vi "anchor map.vi"(11 "string":string) -> (1 "Archt Map":variant, 3 "Lines":string[](array[string]))   [LabVIEW 2020, in "CSMStand-Engine(Lite).lvlib"]
uses:
  CSMStand-Engine(Lite).lvlib
  <userlib>/_NEVSTOP/Communicable State Machine(CSM)/_Shared/CSM Shared.lvlib
  <userlib>/_NEVSTOP/Communicable State Machine(CSM)/Communicable State Machine.lvlib
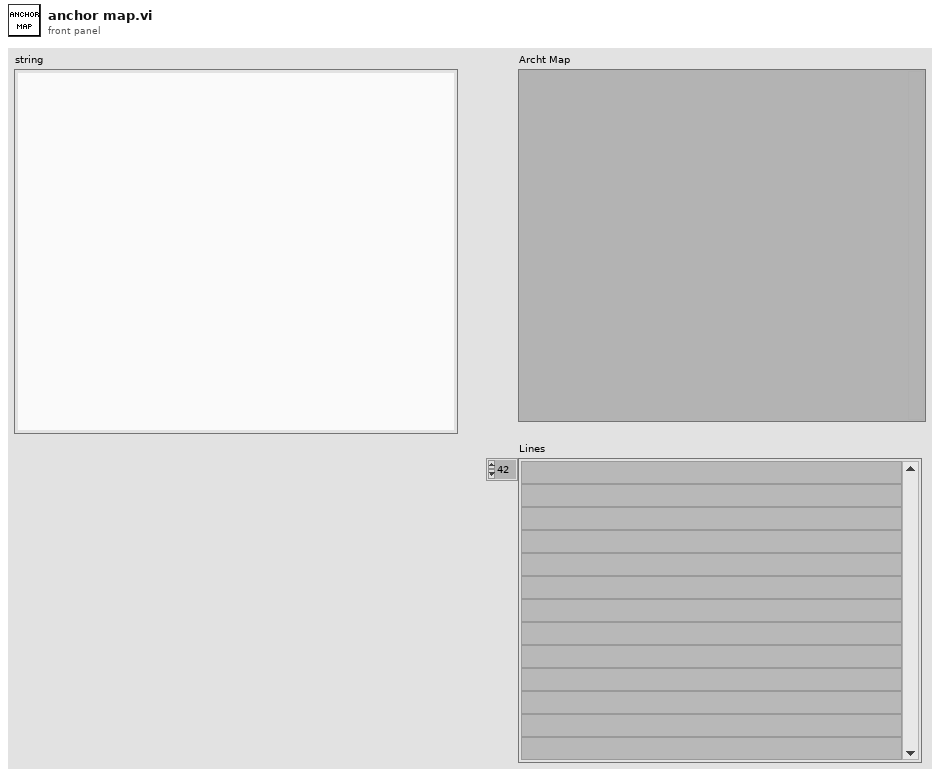
[diagram p1: front panel]
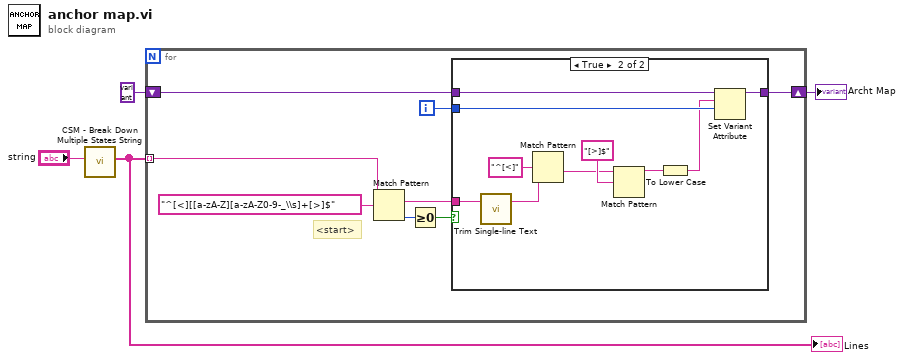
[diagram p0: block diagram]
diagram:
  n1 = call <userlib>:"CSM - Break Down Multiple States String.vi"("States"="string") -> ("Multiple States"=w4:string[])  [unwired: 10 in]
  "Lines" <- w4
  n2 = for {
    tunnel: w4 -> [w12] mode=indexing
    shift-right: [w6] -> w1
    shift-left: variant -> [w7]
    i -> [w5]
    # "<start>"
    n3 = Match Pattern(string=w12, regular expression="^[<][[a-zA-Z][a-zA-Z0-9-_\\s]+[>]$") -> (match substring=w8:string, offset past match=w10:i32)  [unwired: 1 in, 2 out]
    n4 = Greater Or Equal To 0?(x=w10) -> (x >= 0?=w9:bool)
    n5 = case shown="True" w9 {
      tunnel: w7 -> [w13 w23]
      tunnel: [w13 w22] -> w6
      tunnel: w8 -> [_ w21]
      tunnel: w5 -> [_ w16]
      frame False {
      }
      frame True {
        n6 = call <userlib>:"Trim Single-line Text.vi"("single-line text"=w21) -> ("trimed text"=w15:string)  [unwired: 2 in]
        n7 = Match Pattern(string=w15, regular expression="^[<]") -> (after substring=w18:string)  [unwired: 1 in, 3 out]
        n8 = Match Pattern(string=w18, regular expression="[>]$") -> (before substring=w17:string)  [unwired: 1 in, 3 out]
        n9 = To Lower Case(string=w17) -> (all lower case string=w14:string)
        n10 = Set Variant Attribute(Variant=w23, name=w14, value=w16) -> (Variant out=w22:variant)  [unwired: 1 in, 2 out]
      }
    }
  }
  "Archt Map" <- w1
